vi "Write  Input Range (Res).vi"(8 "error in (no error)":errorcluster, 10 "Input Range (Res)":dbl=10.0 format="%#_10g", 11 "ElectrometerInternalConfiguration in":refnum<class "ElectrometerInternalConfiguration.lvclass">) -> (0 "error out":errorcluster, 3 "ElectrometerInternalConfiguration out":refnum<class "ElectrometerInternalConfiguration.lvclass">)   [LabVIEW 2016, in "ElectrometerInternalConfiguration.lvclass"]
uses:
  ElectrometerInternalConfiguration.lvclass
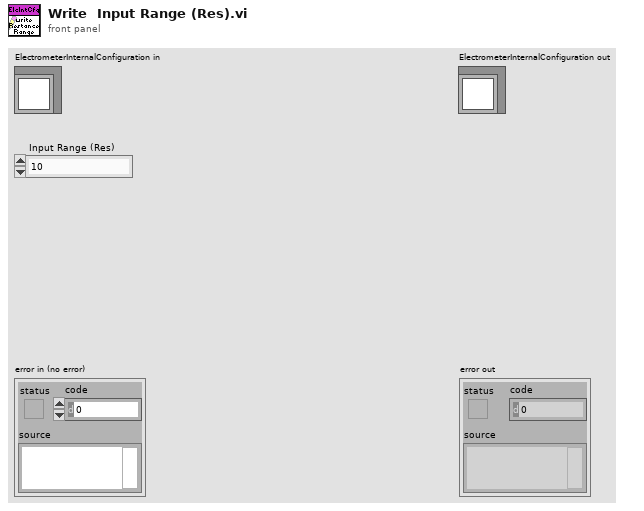
[diagram p1: front panel]
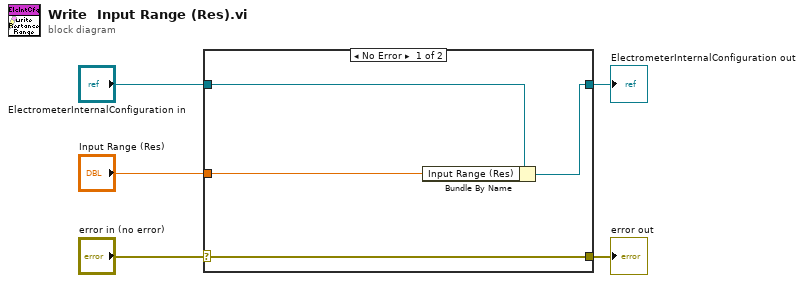
[diagram p0: block diagram]
diagram:
  n1 = case shown="No Error" "error in (no error)" {
    selector: "error in (no error)" -> [w9 w10]
    tunnel: [w9 w10] -> w4
    tunnel: [w7 w11] -> w2
    tunnel: "ElectrometerInternalConfiguration in" -> [w8 w11]
    tunnel: "Input Range (Res)" -> [w6 _]
    frame No Error {
      n2 = Bundle By Name(cluster=w8, "Input Range (Res)"=w6) -> (w7:refnum<class "ElectrometerInternalConfiguration.lvclass">)
    }
    frame Error {
    }
  }
  "error out" <- w4
  "ElectrometerInternalConfiguration out" <- w2
